vi "Auto Loop 0.vi"(2 "Auto State":u8, 3 "Call Context":T1) -> (0 "Loop 0 Data":T2, 1 "SubState 0":T3=enum."driver control")   [LabVIEW 2013]
uses:
  typedefs/subStates.ctl
  typedefs/Loop Datatypes/Loop 0 Datatype.ctl
  <vilib>/Rock Robotics/WPI/DriverStation/WPI_DriverStationDerivedRobotMode.ctl
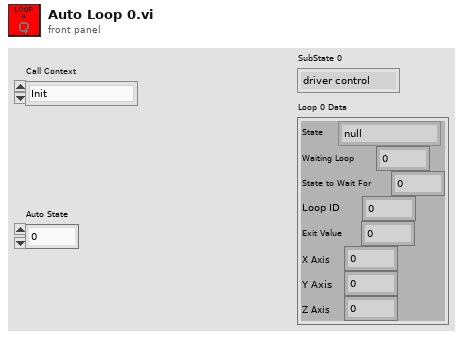
[diagram p1: front panel]
types:
  T1 = typedef "WPI_DriverStationDerivedRobotMode.ctl" = enum16{"Init", "Execute", "Stop"}
  T2 = typedef "Loop 0 Datatype.ctl" = cluster{"State":T3, "Waiting Loop":i32, "State to Wait For":i32, "Loop ID":i32, "Exit Value":i32, "X Axis":dbl, "Y Axis":dbl, "Z Axis":dbl}
  T3 = typedef "subStates.ctl" = enum16{"null", "wait", "driver control", "auto", "manual override", "hold position", "rotate", "pickup", "pass", "load", "goto shoot", "shoot high goal", "shoot low goal", "cancel arm", "cancel shooter", "end", "test"}
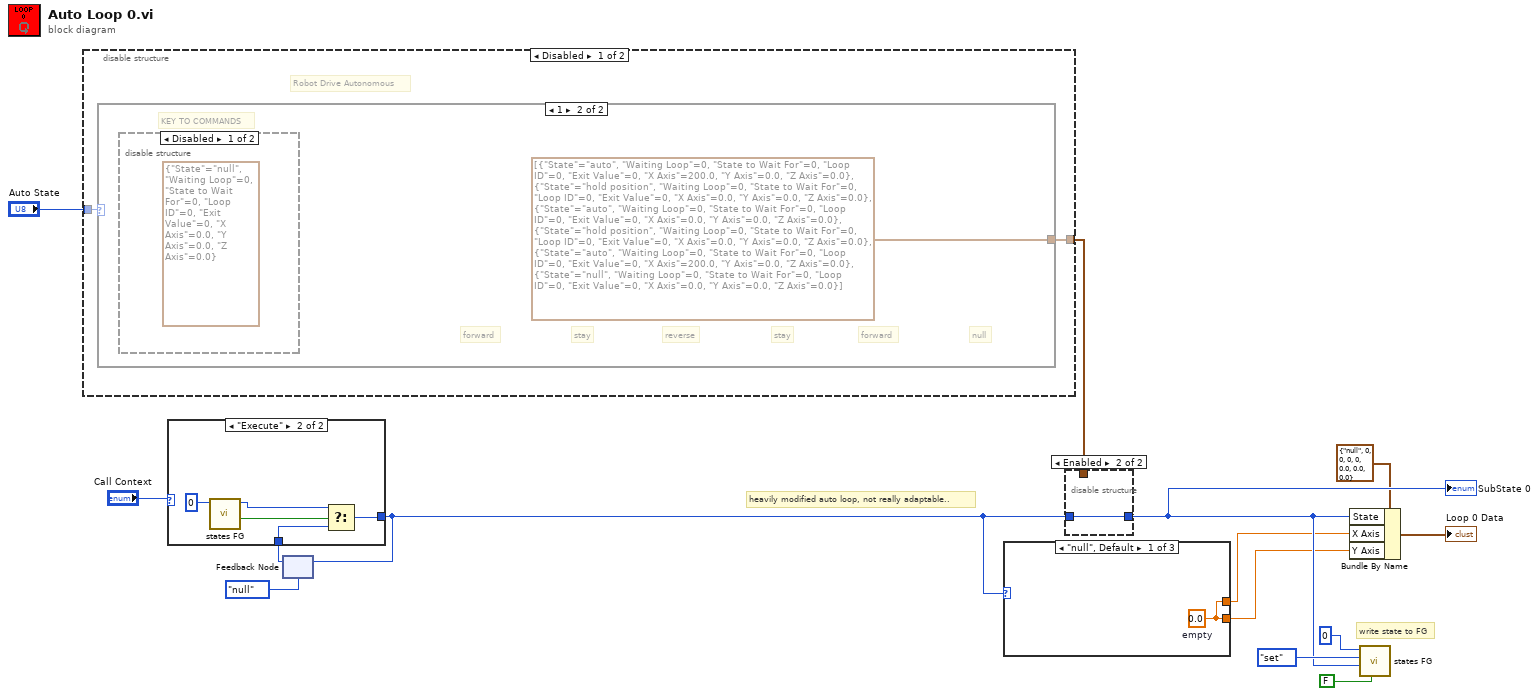
[diagram p0: block diagram]
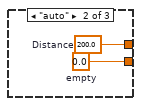
[diagram p2: hidden frame]
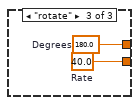
[diagram p3: hidden frame]
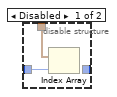
[diagram p4: hidden frame]
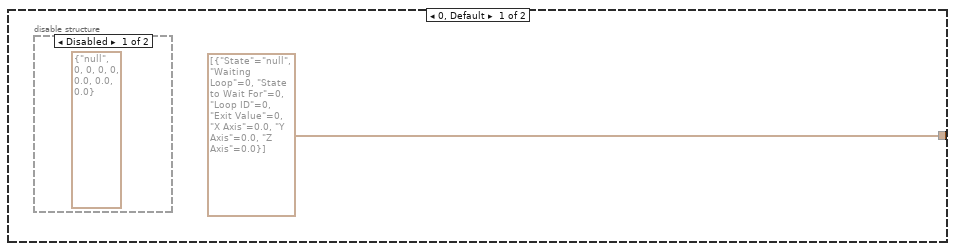
[diagram p5: hidden frame]
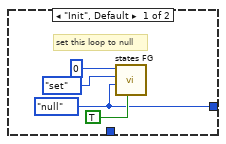
[diagram p9: hidden frame]
diagram:
  # "heavily modified auto loop, not really adaptable.."
  # "write state to FG"
  n1 = disable-structure shown="Disabled" {
    disable-tunnel: "Auto State" -> [w16 _]
    disable-tunnel: [w15 _] -> w11
    frame Disabled {
      # "Robot Drive Autonomous"
      n2 = case shown="1" w16 {
        tunnel: [T2[] [{"State"=enum."null", "Waiting Loop"=0, "State to Wait For"=0, "Loop ID"=0, "Exit Value"=0, "X Axis"=0.0, "Y Axis"=0.0, "Z Axis"=0.0}] T2[] [{"State"=enum."auto", "Waiting Loop"=0, "State to Wait For"=0, "Loop ID"=0, "Exit Value"=0, "X Axis"=200.0, "Y Axis"=0.0, "Z Axis"=0.0}, {"State"=enum."hold position", "Waiting Loop"=0, "State to Wait For"=0, "Loop ID"=0, "Exit Value"=0, "X Axis"=0.0, "Y Axis"=0.0, "Z Axis"=0.0}, {"State"=enum."auto", "Waiting Loop"=0, "State to Wait For"=0, "Loop ID"=0, "Exit Value"=0, "X Axis"=0.0, "Y Axis"=0.0, "Z Axis"=0.0}, {"State"=enum."hold position", "Waiting Loop"=0, "State to Wait For"=0, "Loop ID"=0, "Exit Value"=0, "X Axis"=0.0, "Y Axis"=0.0, "Z Axis"=0.0}, {"State"=enum."auto", "Waiting Loop"=0, "State to Wait For"=0, "Loop ID"=0, "Exit Value"=0, "X Axis"=200.0, "Y Axis"=0.0, "Z Axis"=0.0}, {"State"=enum."null", "Waiting Loop"=0, "State to Wait For"=0, "Loop ID"=0, "Exit Value"=0, "X Axis"=0.0, "Y Axis"=0.0, "Z Axis"=0.0}]] -> w15
        frame 0, Default {
          n3 = disable-structure shown="Disabled" {
            frame Disabled {
              (unwired) T2 {"State"=enum."null", "Waiting Loop"=0, "State to Wait For"=0, "Loop ID"=0, "Exit Value"=0, "X Axis"=0.0, "Y Axis"=0.0, "Z Axis"=0.0} ("Loop 0 Data")
            }
            frame Enabled {
            }
          }
        }
        frame 1 {
          # "null"
          # "forward"
          # "stay"
          # "reverse"
          # "stay"
          # "forward"
          # "KEY TO COMMANDS"
          n4 = disable-structure shown="Disabled" {
            frame Disabled {
              (unwired) T2 {"State"=enum."null", "Waiting Loop"=0, "State to Wait For"=0, "Loop ID"=0, "Exit Value"=0, "X Axis"=0.0, "Y Axis"=0.0, "Z Axis"=0.0} ("Loop 0 Data")
            }
            frame Enabled {
            }
          }
        }
      }
    }
    frame Enabled {
    }
  }
  n5 = feedback #1(subStates."null" ("subState out")) -> (w12:T3)
  n6 = case shown="\"Execute\"" "Call Context" {
    tunnel: w12 -> [_ w26]
    tunnel: [w19 w25] -> w2
    frame "Init", Default {
      w19 = subStates."null" ("subState in")
      # "set this loop to null"
      n7 = call "states FG.vi"("exit in"=TRUE, "subState in"=w19, "menu (get)"=enum16{"set", "get"}."set", "Loop ID"=0) -> ()  [unwired: 4 in, 4 out]
    }
    frame "Execute" {
      n8 = call "states FG.vi"("Loop ID"=0) -> ("exit out"=w24:bool, "subState out"=w23:T3)  [unwired: 7 in, 2 out]
      n9 = Select(t=w23, s=w24, f=w26) -> (s? t:f=w25:T3)
    }
  }
  n10 = feedback-in #1(w2) -> ()
  n11 = case shown="\"null\", Default" w2 {
    tunnel: [w28 w30 w32] -> w3
    tunnel: [w28 w29 w31] -> w1
    frame "null", Default {
      w28 = 0.0  # empty
    }
    frame "auto" {
      w29 = 0.0  # empty
      w30 = 200.0  # Distance
    }
    frame "rotate" {
      w31 = 40.0  # Rate
      w32 = 180.0  # Degrees
    }
  }
  n12 = disable-structure shown="Enabled" {
    disable-tunnel: w11 -> [w34 _]
    disable-tunnel: w2 -> [w33 w35]
    disable-tunnel: [_ w35] -> w6
    frame Disabled {
      n13 = Index Array(array=w34, index=w33) -> ()  [unwired: 1 out]
    }
    frame Enabled {
    }
  }
  "SubState 0" <- w6
  n14 = Bundle By Name(cluster=T2 {"State"=enum."null", "Waiting Loop"=0, "State to Wait For"=0, "Loop ID"=0, "Exit Value"=0, "X Axis"=0.0, "Y Axis"=0.0, "Z Axis"=0.0} ("Loop 0 Data 2"), "State"=w6, "X Axis"=w3, "Y Axis"=w1) -> (→"Loop 0 Data":T2)
  n15 = call "states FG.vi"("exit in"=FALSE, "subState in"=w6, "menu (get)"=enum16{"set", "get"}."set", "Loop ID"=0) -> ()  [unwired: 4 in, 4 out]
